vi "MeasureMeter.vi"(8 "Error In":errorcluster, 11 "VISA resource name":refnum<visa-resource-name>) -> (0 "Error Out":errorcluster, 2 "Meter":T1, 3 "VISA resource name out":refnum<visa-resource-name>)   [LabVIEW 2013]
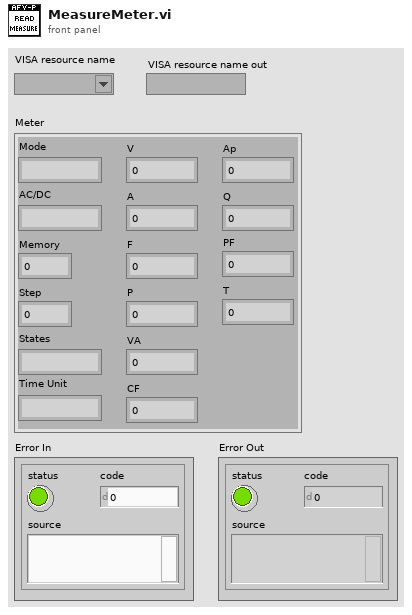
[diagram p1: front panel]
types:
  T1 = cluster{"Mode":string, "AC/DC":string, "Memory":dbl, "Step":dbl, "States":string, "Time Unit":string, "V":dbl, "A":dbl, "F":dbl, "P":dbl, "VA":dbl, "CF":dbl, "Ap":dbl, "Q":dbl, "PF":dbl, "T":dbl}
  T2 = cluster{string, string, i32, i32, string, string, dbl, dbl, dbl, dbl, dbl, dbl, dbl, dbl, dbl, dbl}
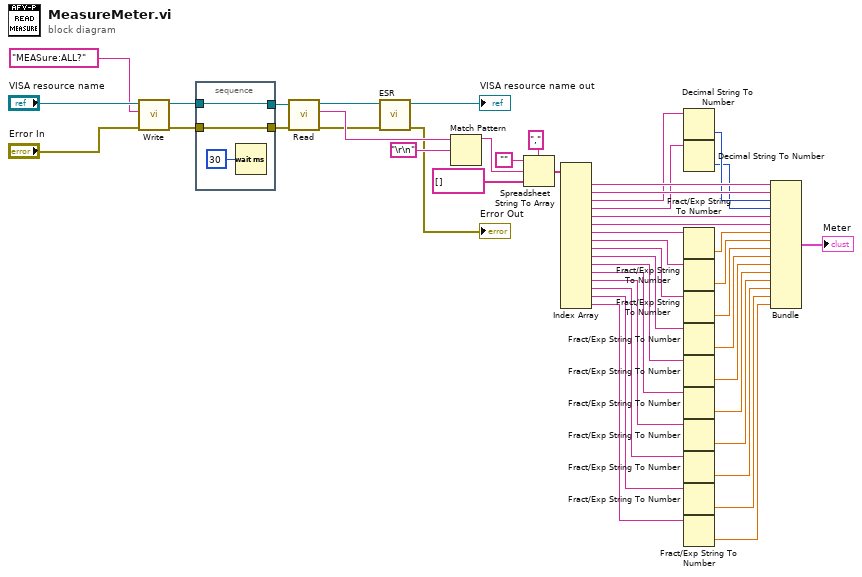
[diagram p0: block diagram]
diagram:
  n1 = call "Write.vi"("Error In"="Error In", "Write Buffer"="MEASure:ALL?", "VISA resource name"="VISA resource name") -> ("Error Out"=w10:errorcluster, "VISA resource name out"=w13:refnum<visa-resource-name>)  [unwired: 7 in]
  n2 = stacked-sequence {
    tunnel: [w49] -> w12
    tunnel: w13 -> [w49]
    tunnel: [w48] -> w11
    tunnel: w10 -> [w48]
    frame #0 {
      n3 = Wait (ms)(milliseconds to wait=u32 30) -> ()  [unwired: 1 out]
    }
  }
  n4 = call "Read.vi"("Error In"=w11, "VISA resource name"=w12) -> ("Error Out"=w8:errorcluster, "Read Data"=w9:string, "VISA resource name out"=w7:refnum<visa-resource-name>)  [unwired: 7 in]
  n5 = call "ESR.vi"("Error In"=w8, "VISA resource name"=w7) -> ("Error Out"=→"Error Out":errorcluster, "VISA resource name out"=→"VISA resource name out":refnum<visa-resource-name>)  [unwired: 8 in]
  n6 = Match Pattern(string=w9, regular expression="\r\n") -> (before substring=w3:string)  [unwired: 1 in, 3 out]
  n7 = Spreadsheet String To Array(delimiter (Tab)=",", format string="", spreadsheet string=w3, array type (2D Dbl)=string[] []) -> (array=w44:string[])
  n8 = Index Array(array=w44) -> (element #1=w43:string, element #2=w42:string, element #3=w41:string, element #4=w40:string, element #5=w37:string, element #6=w36:string, element #7=w35:string, element #8=w34:string, element #9=w33:string, element #10=w32:string, element #11=w31:string, element #12=w30:string, element #13=w29:string, element #14=w15:string, element #15=w28:string, element #16=w27:string)  [unwired: 16 in]
  n9 = Decimal String To Number(string=w41) -> (number=w39:i32)  [unwired: 2 in, 1 out]
  n10 = Decimal String To Number(string=w40) -> (number=w38:i32)  [unwired: 2 in, 1 out]
  n11 = Fract/Exp String To Number(string=w35) -> (number=w26:dbl)  [unwired: 3 in, 1 out]
  n12 = Fract/Exp String To Number(string=w34) -> (number=w25:dbl)  [unwired: 3 in, 1 out]
  n13 = Fract/Exp String To Number(string=w33) -> (number=w24:dbl)  [unwired: 3 in, 1 out]
  n14 = Fract/Exp String To Number(string=w32) -> (number=w23:dbl)  [unwired: 3 in, 1 out]
  n15 = Fract/Exp String To Number(string=w31) -> (number=w22:dbl)  [unwired: 3 in, 1 out]
  n16 = Fract/Exp String To Number(string=w30) -> (number=w21:dbl)  [unwired: 3 in, 1 out]
  n17 = Fract/Exp String To Number(string=w29) -> (number=w20:dbl)  [unwired: 3 in, 1 out]
  n18 = Fract/Exp String To Number(string=w15) -> (number=w19:dbl)  [unwired: 3 in, 1 out]
  n19 = Fract/Exp String To Number(string=w28) -> (number=w18:dbl)  [unwired: 3 in, 1 out]
  n20 = Fract/Exp String To Number(string=w27) -> (number=w17:dbl)  [unwired: 3 in, 1 out]
  n21 = Bundle(w43, w42, w39, w38, w37, w36, w26, w25, w24, w23, w22, w21, w20, w19, w18, w17) -> (→"Meter":T2)  [unwired: 1 in]
